vi "test_joy-sel-axis.vi"(8 "error in":errorcluster, 9 "invert":bool, 10 "select axis":T1, 11 "axis info":T2) -> (0 "error out":errorcluster, 3 "x":dbl)   [LabVIEW 2021]
uses:
  Ctrl/joy-axis.ctl
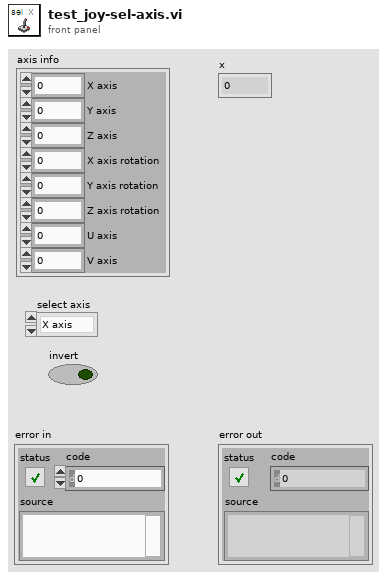
[diagram p1: front panel]
types:
  T1 = typedef "joy-axis.ctl" = enum16{"X axis", "Y axis", "Z axis", "X rotation", "Y rotation", "Z rotation", "U axis", "V axis"}
  T2 = cluster{"X axis":i32, "Y axis":i32, "Z axis":i32, "X axis rotation":i32, "Y axis rotation":i32, "Z axis rotation":i32, "U axis":i32, "V axis":i32}
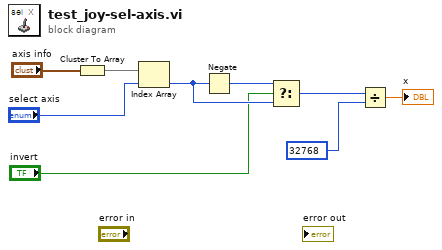
[diagram p0: block diagram]
diagram:
  n1 = Cluster To Array(cluster="axis info") -> (array=w8:i32[])
  n2 = Index Array(array=w8, index="select axis") -> (element=w6:i32)
  n3 = Negate(x=w6) -> (-x=w4:i32)
  n4 = Select(t=w4, s="invert", f=w6) -> (s? t:f=w3:i32)
  n5 = Divide(x=w3, y=32768) -> (x/y=→"x":dbl)
